vi "Disconnect.vi"(8 "error in (no error)":errorcluster, 11 "Network Actor in":refnum<class "Client LNA.lvclass">) -> (0 "error out":errorcluster, 3 "Network Actor out":refnum<class "Client LNA.lvclass">)   [LabVIEW 2016, in "Client LNA.lvlib" / "Client LNA.lvclass"]
doc: "If the local writer stream is connected, flushes the message queue. Destroys the local writer stream."
uses:
  Client LNA.lvclass
  C:/Program Files (x86)/National Instruments/LabVIEW 2016/vi.lib/ActorFramework/Actor/Actor.lvclass
  <vilib>/ActorFramework/Actor/Actor.lvclass/Actor.ctl
  <vilib>/ActorFramework/Message Enqueuer/Message Enqueuer.lvclass/Message Enqueuer.ctl
  <vilib>/ActorFramework/Message Enqueuer/Init from Existing Queue.vi
  <vilib>/ActorFramework/Message Enqueuer/Enqueue.vi
  <vilib>/ActorFramework/Stop Msg/Stop Msg.lvclass
  C:/Program Files (x86)/National Instruments/LabVIEW 2016/vi.lib/ActorFramework/Message/Message.lvclass
  <vilib>/ActorFramework/Message Priority Queue/Priority Enqueue.vi
  <vilib>/NI/Actors/Linked Network Actor/Linked Network Actor/Linked Network Actor.lvclass
  <vilib>/ActorFramework/Message Enqueuer/Message Enqueuer.lvclass
  <vilib>/ActorFramework/Actor/Actor.lvclass
  MAL-Framework/user.lib/Common Components/Controller/Messages/Log Status/Log Status.lvclass
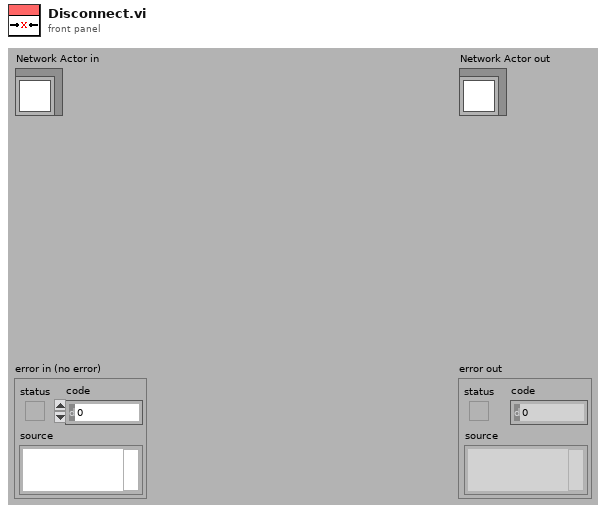
[diagram p1: front panel]
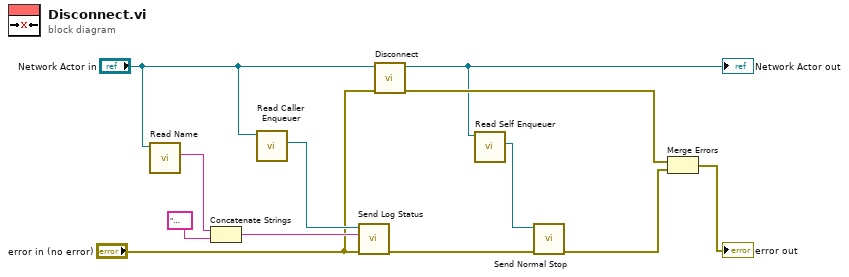
[diagram p0: block diagram]
diagram:
  n1 = call-dynamic "Read Name.vi"("Network Actor in"="Network Actor in") -> ("Name"=w10:string)  [unwired: 10 in]
  n2 = Concatenate Strings(w10, " disconnected" ("string")) -> (w11:string)
  n3 = call <vilib>:"Read Caller Enqueuer.vi"("Actor"="Network Actor in") -> ("Caller Enqueuer"=w12:refnum<class "Message Enqueuer.lvclass">)  [unwired: 10 in]
  n4 = call "Send Log Status.vi"("error in (no error)"="error in (no error)", "String"=w11, "Message Enqueuer in"=w12) -> ("error out"=w7:errorcluster)  [unwired: 7 in, 1 out]
  n5 = call-parent "Disconnect.vi"("error in (no error)"="error in (no error)", "Network Actor in"="Network Actor in") -> ("error out"=w6:errorcluster, "Network Actor out"=w3:refnum<class "Client LNA.lvclass">)  [unwired: 8 in]
  "Network Actor out" <- w3
  n6 = call <vilib>:"Read Self Enqueuer.vi"("Actor"=w3) -> ("Self Enqueuer"=w2:refnum<class "Message Enqueuer.lvclass">)  [unwired: 10 in]
  n7 = call <vilib>:"Send Normal Stop.vi"("error in (no error)"=w7, "Message Enqueuer"=w2) -> ("error out"=w4:errorcluster)  [unwired: 9 in]
  n8 = Merge Errors(w6, w4) -> (→"error out":errorcluster)
